vi "TestExec.Get Limit File.vi"(8 "error in (no error)":errorcluster, 11 "Folder":path) -> (0 "error out":errorcluster, 1 "Version":string, 2 "Name":string, 3 "Path":path)   [LabVIEW 2018]
uses:
  <vilib>/KATE/Files/File Utils.lvlib
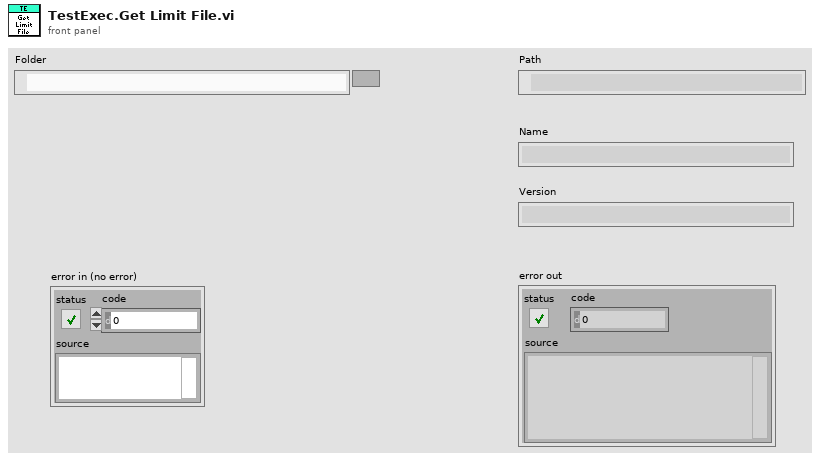
[diagram p1: front panel]
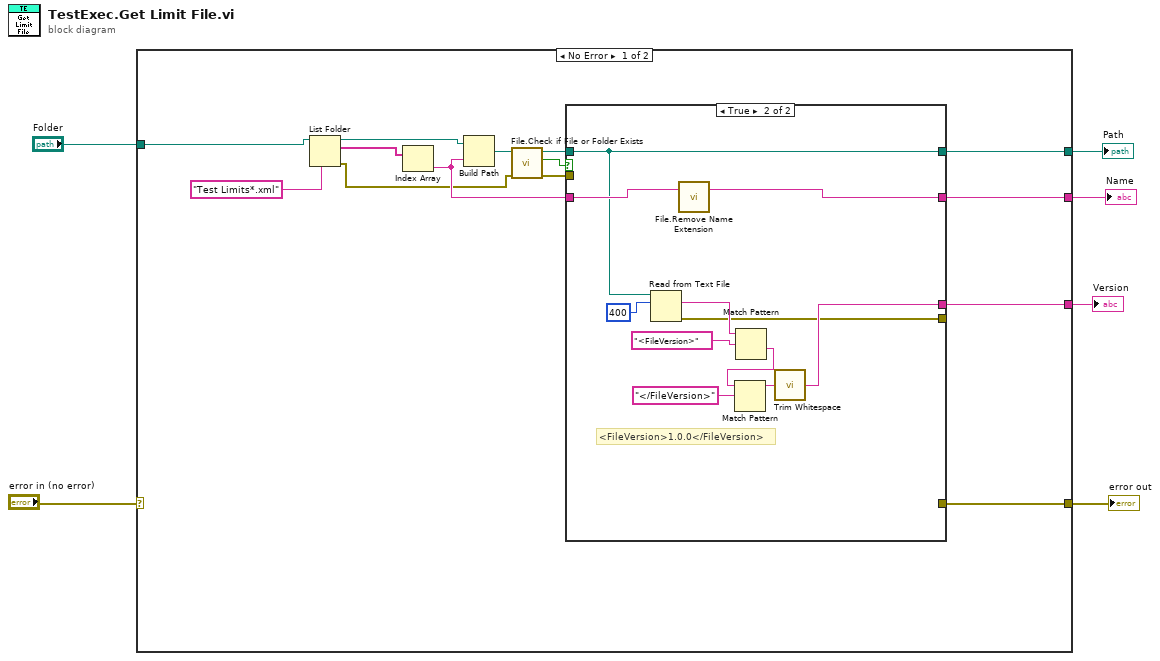
[diagram p0: block diagram]
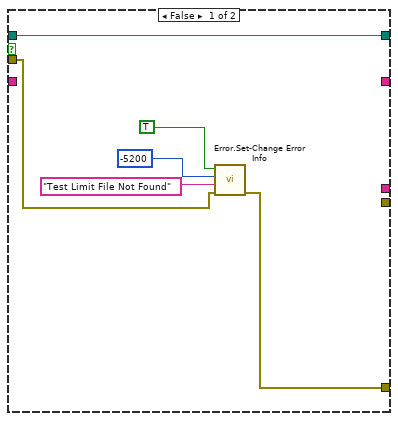
[diagram p2: hidden frame]
diagram:
  n1 = case shown="No Error" "error in (no error)" {
    selector: "error in (no error)" -> [_ w38]
    tunnel: "Folder" -> [w7 _]
    tunnel: [w17 _] -> w5
    tunnel: [w11 _] -> w4
    tunnel: [w15 _] -> w3
    tunnel: [w9 w38] -> w1
    frame No Error {
      n2 = List Folder(path=w7, pattern="Test Limits*.xml") -> (path out=w18:path, filenames=w19:string[], error out=w12:errorcluster)  [unwired: 2 in, 1 out]
      n3 = Index Array(array=w19) -> (element=w14:string)  [unwired: 1 in]
      n4 = Build Path(base path=w18, name or relative path=w14) -> (appended path=w13:path)
      n5 = call <vilib>:"File.Check if File or Folder Exists.vi"("error in"=w12, "Path"=w13) -> ("error out"=w8:errorcluster, "Exists"=w10:bool, "Dup Path"=w16:path)  [unwired: 5 in, 2 out]
      n6 = case shown="True" w10 {
        tunnel: [_ w37] -> w17
        tunnel: w16 -> [w26 w28]
        tunnel: [_ w36] -> w15
        tunnel: w14 -> [_ w35]
        tunnel: [w26 w28] -> w11
        tunnel: [w25 _] -> w9
        tunnel: w8 -> [w21 _]
        tunnel: [_ w27] -> _
        frame False {
          n7 = call "Error.Set-Change Error Info.vi"("error in"=w21, "Description"="Test Limit File Not Found", "Cust Code(0 = no change)"=-5200 ("Code(0 = no change)"), "Set Error"=TRUE) -> ("error out"=w25:errorcluster)  [unwired: 7 in]
        }
        frame True {
          # "<FileVersion>1.0.0</FileVersion>"
          n8 = Read from Text File(file (use dialog)=w28, count=400) -> (text=w34:string, error out=w27:errorcluster)  [unwired: 2 in, 2 out]
          n9 = call <vilib>:"File.Remove Name Extension.vi"("File Name"=w35) -> ("Name Less Ext"=w37:string)  [unwired: 1 in, 1 out]
          n10 = Match Pattern(string=w34, regular expression="<FileVersion>") -> (after substring=w30:string)  [unwired: 1 in, 3 out]
          n11 = Match Pattern(string=w30, regular expression="</FileVersion>") -> (before substring=w29:string)  [unwired: 1 in, 3 out]
          n12 = call <vilib>:"Trim Whitespace.vi"("string"=w29) -> ("trimmed string"=w36:string)  [unwired: 1 in]
        }
      }
    }
    frame Error {
    }
  }
  "Name" <- w5
  "Version" <- w3
  "Path" <- w4
  "error out" <- w1
